vi "new imu.vi"(11 "error in (no error)":errorcluster) -> (0 "Numeric":dbl format="%#_13g", 3 "error out":errorcluster)   [LabVIEW 2015]
uses:
  <vilib>/myRIO/Instrument Drivers/Onboard IO/I2C/typedefs/I2C User Configuration.ctl
  <vilib>/myRIO/Instrument Drivers/Onboard IO/I2C/typedefs/I2C Transfer Rate.ctl
  <vilib>/myRIO/Instrument Drivers/Onboard IO/I2C/typedefs/I2C Reference.ctl
  <vilib>/myRIO/Common/Instrument Driver Framework/Utilities/typedefs/myRIO Generic Hardware Reference.ctl
  <vilib>/myRIO/Common/Instrument Driver Framework/Utilities/typedefs/Hardware Version Enum.ctl
  <vilib>/myRIO/Common/Instrument Driver Framework/Utilities/typedefs/myRIO v1.0 Reference.ctl
  <vilib>/myRIO/Common/Instrument Driver Framework/Utilities/typedefs/Generic FPGA Reference.ctl
  <vilib>/myRIO/Common/Instrument Driver Framework/myRIO v1.0/I2C/typedefs/I2C Channels Enum.ctl
  <vilib>/myRIO/Instrument Drivers/Onboard IO/I2C/typedefs/I2C Configuration.ctl
  <vilib>/userdefined/High Color/nirio_resource_hc.ctl
  <vilib>/myRIO/Common/Instrument Driver Framework/Utilities/vis/Is FPGA Ref Available.vi
  <vilib>/myRIO/Common/Instrument Driver Framework/myRIO v1.0/I2C/vis/myRIO v1.1 Open I2C.vi
  <vilib>/myRIO/Instrument Drivers/Onboard IO/I2C/vis/Configure.vi
  <vilib>/myRIO/Instrument Drivers/Onboard IO/I2C/vis/Write.vi
  <vilib>/myRIO/Instrument Drivers/Onboard IO/I2C/vis/Read.vi
  <vilib>/myRIO/Common/Instrument Driver Framework/Utilities/vis/Validate Channels.vi
  <vilib>/myRIO/Common/Instrument Driver Framework/myRIO v1.0/I2C/vis/myRIO v1.0 Reserve I2C.vi
  <vilib>/myRIO/Common/Instrument Driver Framework/myRIO v1.0/I2C/vis/myRIO v1.0 Build MUX Configuration I2C.vi
  <vilib>/myRIO/Common/Instrument Driver Framework/myRIO v1.0/Resource Manager/vis/myRIO v1.0 Reserve Channel List.vi
  <vilib>/myRIO/Common/Instrument Driver Framework/myRIO v1.0/Resource Manager/vis/myRIO v1.0 Create Configuration List.vi
  <vilib>/myRIO/Common/Instrument Driver Framework/myRIO v1.0/Resource Manager/vis/myRIO v1.0 Reserve Channel.vi
  <vilib>/myRIO/Common/Instrument Driver Framework/myRIO v1.0/Resource Manager/vis/myRIO v1.0 Unreserve Channel.vi
  <vilib>/myRIO/Common/Instrument Driver Framework/myRIO v1.0/Resource Manager/vis/myRIO v1.0 Build Mutex Name.vi
  <vilib>/Utility/VariantDataType/GetNumericInfo.vi
  <vilib>/Utility/error.llb/Error Cluster From Error Code.vi
  <vilib>/myRIO/Common/Instrument Driver Framework/myRIO v1.0/myRIO v1.1 Open.vi
  <vilib>/myRIO/Common/Instrument Driver Framework/Utilities/vis/IO Manager.vi
  <vilib>/myRIO/Common/Instrument Driver Framework/Utilities/vis/Configuration Manager.vi
  <vilib>/myRIO/Common/Instrument Driver Framework/myRIO v1.0/Resource Manager/vis/myRIO v1.0 Configure IO.vi
  <vilib>/myRIO/Common/Instrument Driver Framework/myRIO v1.0/myRIO v1.0 Close.vi
  <vilib>/myRIO/Common/Instrument Driver Framework/myRIO v1.0/I2C/vis/myRIO v1.0 Configure I2C.vi
  <vilib>/myRIO/Common/Instrument Driver Framework/myRIO v1.0/I2C/vis/myRIO v1.0 Write I2C.vi
  <vilib>/myRIO/Common/Instrument Driver Framework/myRIO v1.0/I2C/vis/myRIO v1.0 Read I2C.vi
  <vilib>/myRIO/Express VI/Onboard IO/I2C/I2C Express VI.xnode
  <vilib>/myRIO/Instrument Drivers/Onboard IO/I2C/vis/myRIO I2C Open.xnode
  <vilib>/myRIO/Instrument Drivers/Onboard IO/I2C/I2C.lvlib
panel:
  out "Heading Data":T1
  out "Array 2":u8[](array[numeric]) format="%b"
  out "Array":u8[](array[numeric]) format="%b"
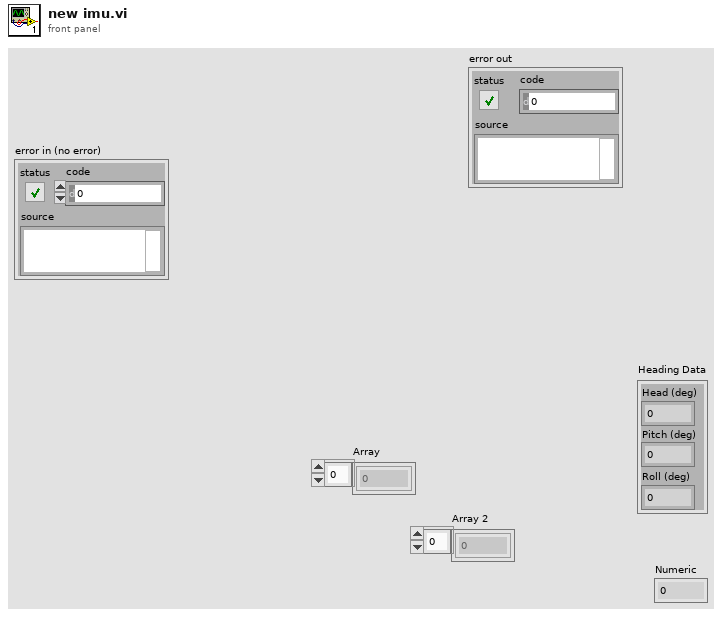
[diagram p1: front panel]
types:
  T1 = cluster{"Head (deg)":dbl, "Pitch (deg)":dbl, "Roll (deg)":dbl}
  T2 = typedef "I2C.lvlib/I2C Reference.ctl" = cluster{"myRIO Reference":T3, "I2C Channels Enum":T7, "I2C Configuration":T8}
  T3 = typedef "myRIO Generic Hardware Reference.ctl" = cluster{"myRIO Model":T4, "myRIO Hardware Reference":T5}
  T4 = typedef "Hardware Version Enum.ctl" = enum16{"Unknown", "myRIO-1900", "myRIO-1950", "roboRIO"}
  T5 = typedef "myRIO v1.0 Reference.ctl" = cluster{"Generic FPGA Reference":T6, "Allow multiple opens":bool}
  T6 = typedef "Generic FPGA Reference.ctl" = refnum<k20>
  T7 = typedef "I2C Channels Enum.ctl" = enum16{"Not Connected", "A/I2C", "B/I2C", "I2C/I2C"}
  T8 = typedef "I2C.lvlib/I2C Configuration.ctl" = cluster{"I2C Transfer Rate":T9}
  T9 = typedef "I2C.lvlib/I2C Transfer Rate.ctl" = enum16{"Standard mode (100 kbps)", "Fast mode (400 kbps)"}
  T10 = typedef "I2C.lvlib/I2C User Configuration.ctl" = cluster{"I2C Transfer Rate":T9}
  T11 = typedef "nirio_resource_hc.ctl" = tag
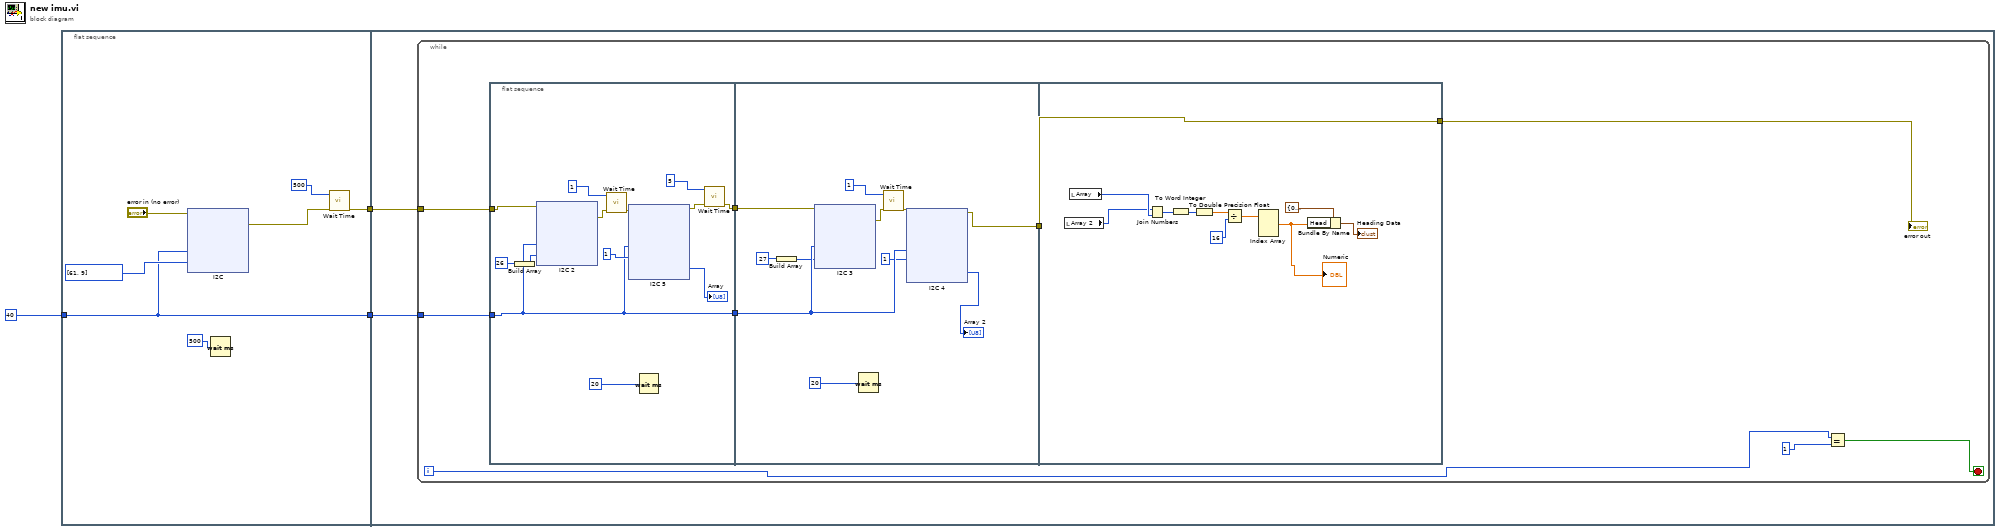
[diagram p0: block diagram]
diagram:
  n1 = flat-sequence {
    tunnel: [w5] -> w3
    tunnel: 40 -> [w4]
    tunnel: [w4] -> w1
    tunnel: w3 -> [w50]
    tunnel: w1 -> [w49]
    frame #0 {
      n2 = xnode "I2C"("Slave Address (7-bit)"=w4, "Bytes to Write"=i32[] [61, 9], "error in (no error)"="error in (no error)") -> ("error out"=w8:errorcluster)
      n3 = Wait (ms)(milliseconds to wait=500) -> ()  [unwired: 1 out]
      n4 = call "Wait Time.vi"("error in (no error)"=w8, "Wait Time (ms)"=500) -> ("error out"=w5:errorcluster)  [unwired: 9 in]
    }
    frame #1 {
      n5 = while {
        tunnel: w50 -> [w55]
        tunnel: w49 -> [w54]
        i -> [w51]
        stop <- w53 stop-if-true
        n6 = flat-sequence {
          tunnel: [w62] -> w59
          tunnel: [w60] -> w58
          tunnel: w55 -> [w61]
          tunnel: w54 -> [w60]
          tunnel: w59 -> [w160]
          tunnel: [w159] -> w57
          tunnel: w58 -> [w158]
          tunnel: w57 -> [w248]
          tunnel: [w248] -> w56
          frame #0 {
            n7 = Build Array(26) -> (w69:i32[])
            n8 = xnode "I2C 2"("Slave Address (7-bit)"=w60, "Bytes to Write"=w69, "error in (no error)"=w61) -> ("error out"=w66:errorcluster)
            n9 = call "Wait Time.vi"("error in (no error)"=w66, "Wait Time (ms)"=1) -> ("error out"=w65:errorcluster)  [unwired: 9 in]
            n10 = xnode "I2C 5"("Slave Address (7-bit)"=w60, "Byte Count"=1, "error in (no error)"=w65) -> ("Bytes Read"=→"Array":u8[], "error out"=w63:errorcluster)
            n11 = Wait (ms)(milliseconds to wait=20) -> ()  [unwired: 1 out]
            n12 = call "Wait Time.vi"("error in (no error)"=w63, "Wait Time (ms)"=5) -> ("error out"=w62:errorcluster)  [unwired: 9 in]
          }
          frame #1 {
            n13 = Build Array(27) -> (w154:i32[])
            n14 = xnode "I2C 3"("Slave Address (7-bit)"=w158, "Bytes to Write"=w154, "error in (no error)"=w160) -> ("error out"=w151:errorcluster)
            n15 = Wait (ms)(milliseconds to wait=20) -> ()  [unwired: 1 out]
            n16 = call "Wait Time.vi"("error in (no error)"=w151, "Wait Time (ms)"=1) -> ("error out"=w150:errorcluster)  [unwired: 9 in]
            n17 = xnode "I2C 4"("Slave Address (7-bit)"=w158, "Byte Count"=1, "error in (no error)"=w150) -> ("Bytes Read"=→"Array 2":u8[], "error out"=w159:errorcluster)
          }
          frame #2 {
            n18 = local read "Array 2"() -> (w238:u8[])
            n19 = local read "Array"() -> (w239:u8[])
            n20 = Join Numbers(hi=w238, lo=w239) -> ((hi.lo)=w245:u16[])
            n21 = To Word Integer(number=w245) -> (16bit integer=w244:i16[])
            n22 = To Double Precision Float(number=w244) -> (double precision float=w243:dbl[])
            n23 = Divide(x=w243, y=16) -> (x/y=w242:dbl[])
            n24 = Index Array(array=w242) -> (element #1=w240:dbl)  [unwired: 3 in, 2 out]
            "Numeric" <- w240
            n25 = Bundle By Name(cluster=cluster{"Head":dbl, "Pitch":dbl, "Roll":dbl} {"Head"=0.0, "Pitch"=0.0, "Roll"=0.0} ("Heading Data"), "Head"=w240) -> (→"Heading Data":cluster{"Head":dbl, "Pitch":dbl, "Roll":dbl})
          }
        }
        n26 = Equal?(x=w51, y=1) -> (x = y?=w53:bool)
        "error out" <- w56
      }
    }
  }
